vi "Calc_rhoplus.vi"(10 "Q":dbl[](array[numeric]), 11 "P":dbl[](array[numeric])) -> (3 "rho+":dbl[](array[numeric]))   [LabVIEW 2018]
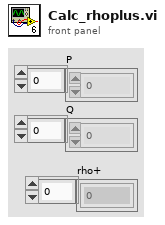
[diagram p1: front panel]
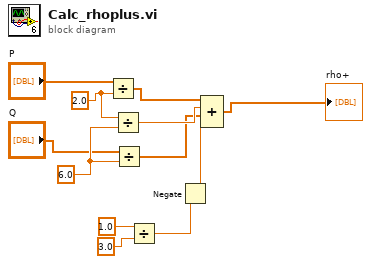
[diagram p0: block diagram]
diagram:
  w10 = 6.0
  w11 = 2.0
  n1 = Divide(x="P", y=w11) -> (x/y=w6:dbl[])
  n2 = Divide(x=w11, y=w10) -> (x/y=w8:dbl)
  n3 = Divide(x="Q", y=w10) -> (x/y=w7:dbl[])
  n4 = Divide(x=1.0, y=3.0) -> (x/y=w2:dbl)
  n5 = Negate(x=w2) -> (-x=w1:dbl)
  n6 = Compound Arithmetic op=ADD(w6, w8, w7, w1) -> (→"rho+":dbl[])
